vi "Get or Add Workbookpart.vi"(8 "error in":errorcluster, 11 "SpreadsheetDoc in":refnum<k24>) -> (0 "error out":errorcluster, 2 "WorkbookPart":refnum<k24>, 3 "SpreadsheetDoc out":refnum<k24>)   [LabVIEW 2019, in "Open Xml.lvlib"]
uses:
  Open Xml.lvlib
  D:/git/Open-Xml-LabVIEW/Source/DocumentFormat.OpenXml.dll
  DocumentFormat.OpenXml.dll
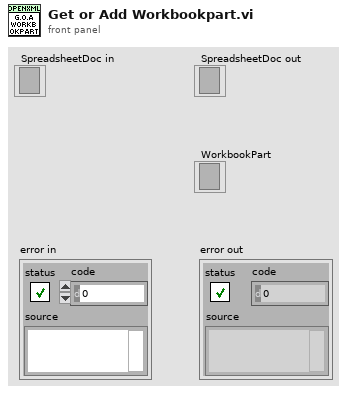
[diagram p1: front panel]
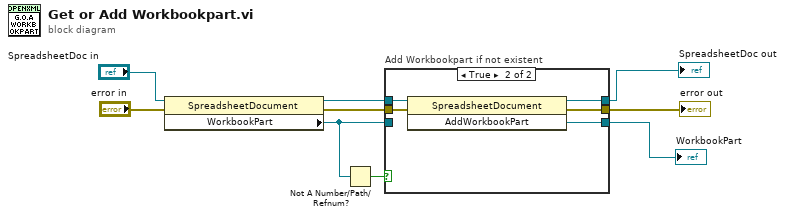
[diagram p0: block diagram]
diagram:
  n1 = property class="SpreadsheetDocument"(reference="SpreadsheetDoc in", error in="error in") -> (reference out=w2:refnum<k24>, error out=w1:errorcluster, "WorkbookPart"=w3:refnum<k24>)
  n2 = Not A Number/Path/Refnum?(number/path/refnum=w3) -> (NaN/Path/Refnum?=w4:bool)
  n3 = case "Add Workbookpart if not existent" shown="True" w4 {
    tunnel: w3 -> [w10 _]
    tunnel: w2 -> [w11 w17]
    tunnel: w1 -> [w12 w16]
    tunnel: [w11 w15] -> w6
    tunnel: [w12 w14] -> w8
    tunnel: [w10 w13] -> w5
    frame False {
    }
    frame True {
      n4 = invoke class="SpreadsheetDocument" method="AddWorkbookPart"(reference=w17, error in=w16) -> (reference out=w15:refnum<k24>, error out=w14:errorcluster, "AddWorkbookPart"=w13:refnum<k24>)  [unwired: 1 in]
    }
  }
  "error out" <- w8
  "SpreadsheetDoc out" <- w6
  "WorkbookPart" <- w5
